vi "GDSProject_SaveProject.vi"(10 "error in (no error)":errorcluster, 11 "Project in":refnum<vi>) -> (2 "error out":errorcluster, 3 "Project out":refnum<vi>)   [LabVIEW 2020]
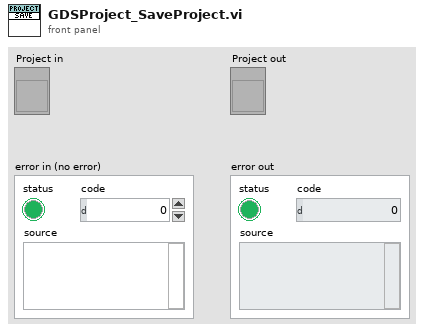
[diagram p1: front panel]
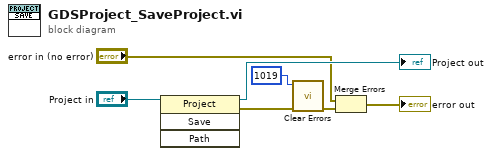
[diagram p0: block diagram]
diagram:
  n1 = invoke class="Project" method="Save"(reference="Project in") -> (reference out=→"Project out":refnum<vi>, error out=w2:errorcluster)  [unwired: 3 in, 2 out]
  n2 = call <vilib>:"Clear Errors.vi"("error in (no error)"=w2, "specific error code to clear (0: all)"=1019) -> ("error out"=w1:errorcluster)  [unwired: 4 in, 1 out]
  n3 = Merge Errors("error in (no error)", w1) -> (→"error out":errorcluster)
